vi "Calculate Average Center.vi"(11 "Gantry Fiducials":dbl[](array[numeric])) -> (1 "Sensor ID Location":dbl[](array[numeric]), 2 "CH1 Location":dbl[](array[numeric]), 3 "XYZTheta":dbl[](array[numeric]))   [LabVIEW 2018, in "Component Tray.lvclass"]
uses:
  Component Tray.lvclass
  <vilib>/Analysis/baseanly.llb/Mean (DBL).vi
  <vilib>/Analysis/NI_AALBase.lvlib
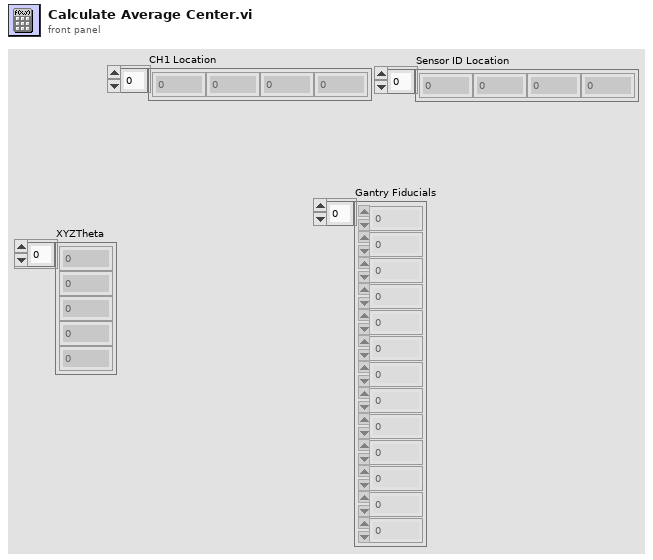
[diagram p1: front panel]
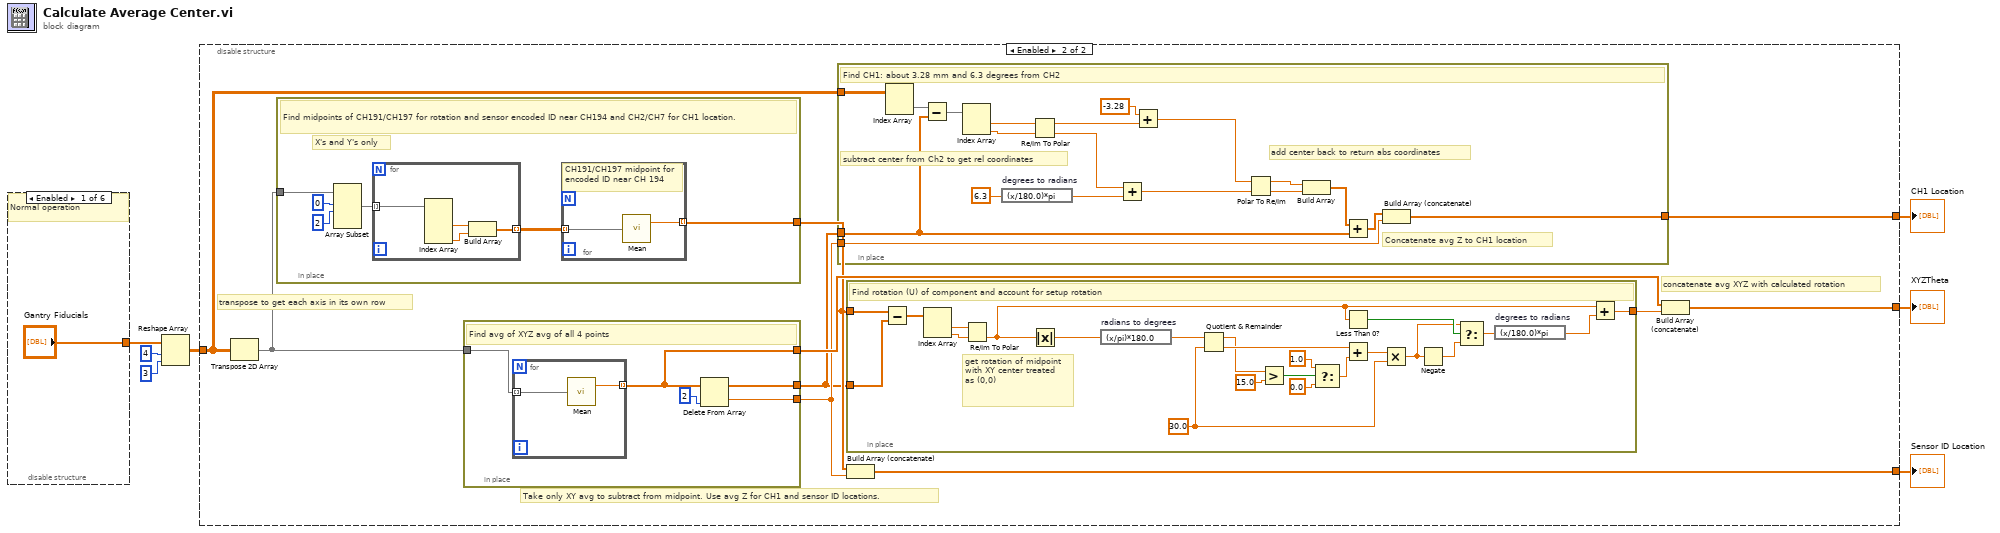
[diagram p0: block diagram]
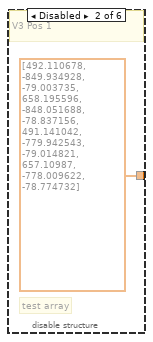
[diagram p2: hidden frame]
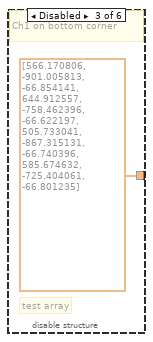
[diagram p3: hidden frame]
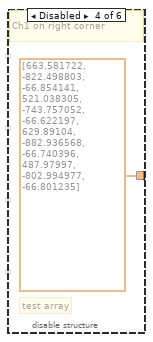
[diagram p4: hidden frame]
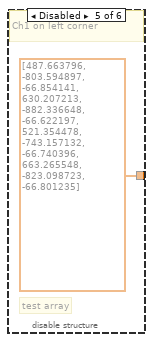
[diagram p5: hidden frame]
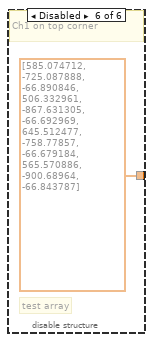
[diagram p6: hidden frame]
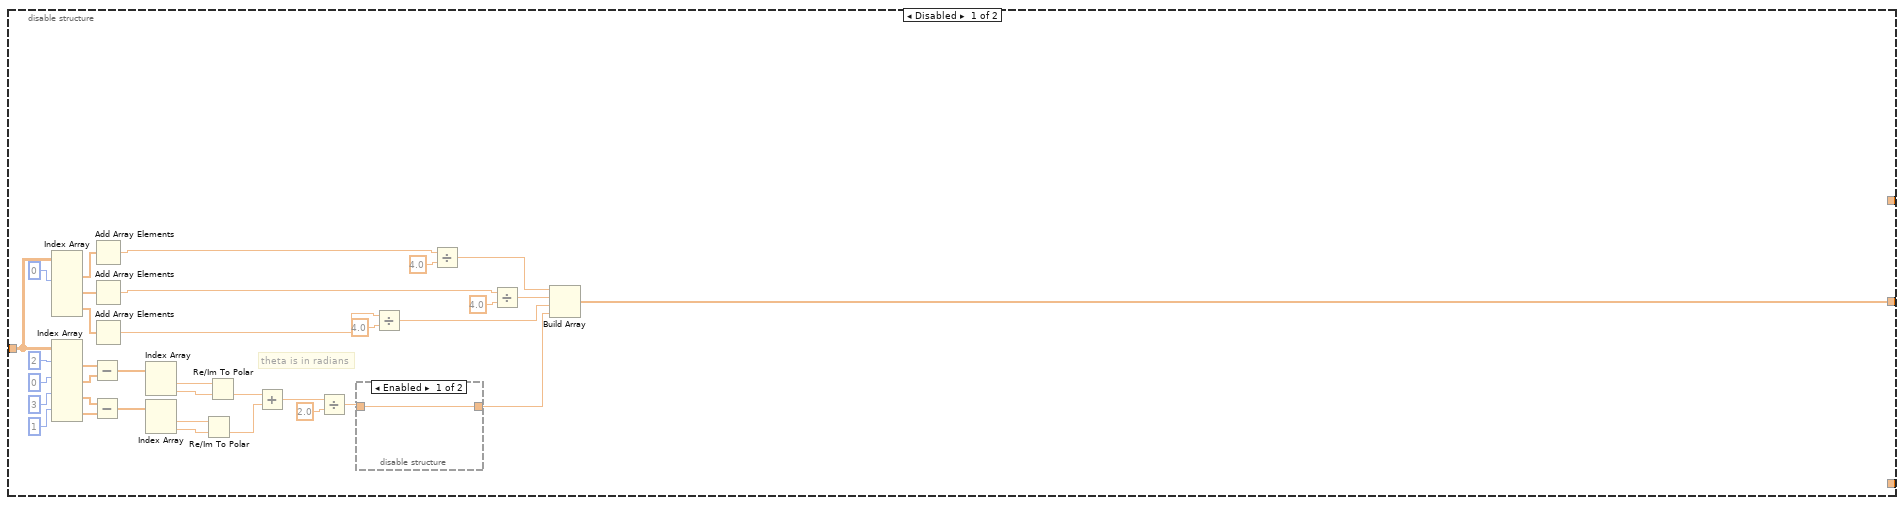
[diagram p7: hidden frame]
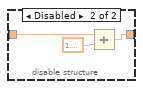
[diagram p8: hidden frame]
diagram:
  n1 = disable-structure shown="Enabled" {
    disable-tunnel: ["Gantry Fiducials" dbl[] [492.110678, -849.934928, -79.003735, 658.195596, -848.051688, -78.837156, 491.141042, -779.942543, -79.014821, 657.10987, -778.009622, -78.774732] dbl[] [566.170806, -901.005813, -66.854141, 644.912557, -758.462396, -66.622197, 505.733041, -867.315131, -66.740396, 585.674632, -725.404061, -66.801235] dbl[] [663.581722, -822.498803, -66.854141, 521.038305, -743.757052, -66.622197, 629.89104, -882.936568, -66.740396, 487.97997, -802.994977, -66.801235] dbl[] [487.663796, -803.594897, -66.854141, 630.207213, -882.336648, -66.622197, 521.354478, -743.157132, -66.740396, 663.265548, -823.098723, -66.801235] dbl[] [585.074712, -725.087888, -66.890846, 506.332961, -867.631305, -66.692969, 645.512477, -758.77857, -66.679184, 565.570886, -900.68964, -66.843787]] -> w6
    frame Enabled {
      # "Normal operation"
    }
    frame Disabled {
      # "test array"
      # "V3 Pos 1"
    }
    frame Disabled {
      # "test array"
      # "Ch1 on bottom corner"
    }
    frame Disabled {
      # "test array"
      # "Ch1 on right corner"
    }
    frame Disabled {
      # "test array"
      # "Ch1 on left corner"
    }
    frame Disabled {
      # "test array"
      # "Ch1 on top corner"
    }
  }
  n2 = Reshape Array(w6, 4 ("dimension size"), 3 ("dimension size")) -> (w3:dbl[][])
  n3 = disable-structure shown="Enabled" {
    disable-tunnel: [w18 w62] -> w7
    disable-tunnel: w3 -> [w17 w53]
    disable-tunnel: [_ w58] -> w5
    disable-tunnel: [_ w61] -> w4
    frame Disabled {
      # "theta is in radians"
      n4 = Index Array(array=w17, index (col) #1=0 ("disabled index (col)")) -> (element #1=w47:dbl[], element #2=w46:dbl[], element #3=w16:dbl[])  [unwired: 5 in]
      n5 = Index Array(array=w17, index (row) #1=2 ("index (row)"), index (row) #2=0 ("index (row)"), index (row) #3=3 ("index (row)"), index (row) #4=1 ("index (row)")) -> (element #1=w31:dbl[], element #2=w30:dbl[], element #3=w29:dbl[], element #4=w28:dbl[])  [unwired: 4 in]
      n6 = Subtract(x=w31, y=w30) -> (x-y=w41:dbl[])
      n7 = Subtract(x=w29, y=w28) -> (x-y=w40:dbl[])
      n8 = Add Array Elements(numeric array=w47) -> (sum=w45:dbl)
      n9 = Add Array Elements(numeric array=w46) -> (sum=w44:dbl)
      n10 = Add Array Elements(numeric array=w16) -> (sum=w22:dbl)
      n11 = Index Array(array=w41) -> (element #1=w39:dbl, element #2=w38:dbl)  [unwired: 2 in]
      n12 = Index Array(array=w40) -> (element #1=w37:dbl, element #2=w36:dbl)  [unwired: 2 in]
      n13 = Re/Im To Polar(2:w36, 3:w37) -> (0:w34:dbl)  [unwired: 1 out]
      n14 = Re/Im To Polar(2:w38, 3:w39) -> (0:w35:dbl)  [unwired: 1 out]
      n15 = Add(x=w35, y=w34) -> (x+y=w33:dbl)
      n16 = Divide(x=w33, y=2.0) -> (x/y=w15:dbl)
      n17 = disable-structure shown="Enabled" {
        disable-tunnel: w15 -> [w49 w51]
        disable-tunnel: [w49 w50] -> w14
        frame Enabled {
        }
        frame Disabled {
          n18 = Add(x=w51, y=1.5707963267948966) -> (x+y=w50:dbl)
        }
      }
      n19 = Divide(x=w22, y=4.0) -> (x/y=w19:dbl)
      n20 = Divide(x=w45, y=4.0) -> (x/y=w21:dbl)
      n21 = Divide(x=w44, y=4.0) -> (x/y=w20:dbl)
      n22 = Build Array(w21, w20, w19, w14) -> (w18:dbl[])
    }
    frame Enabled {
      # "concatenate avg XYZ with calculated rotation"
      # "Take only XY avg to subtract from midpoint. Use avg Z for CH1 and sensor ID locations."
      # "transpose to get each axis in its own row"
      n23 = Transpose 2D Array(2D array=w53) -> (transposed array=w59:dbl[][])
      n24 = in-place {
        in-place-border: w59 -> [w110]
        in-place-border: [w105] -> w56
        # "X's and Y's only"
        # "Find midpoints of CH191/CH197 for rotation and sensor encoded ID near CH194 and CH2/CH7 for CH1 location."
        n25 = Array Subset(array=w110, index (row)=0 ("index"), length (row)=2 ("length")) -> (w107:dbl[][])  [unwired: 2 in]
        n26 = for {
          tunnel: w107 -> [w116] mode=indexing
          tunnel: [w113] -> w106 mode=indexing
          n27 = Index Array(array=w116) -> (element #2=w115:dbl, element #4=w114:dbl)  [unwired: 4 in, 2 out]
          n28 = Build Array(w115, w114) -> (w113:dbl[])
        }
        n29 = for {
          tunnel: [w111] -> w105 mode=indexing
          tunnel: w106 -> [w112] mode=indexing
          # "CH191/CH197 midpoint for encoded ID near CH 194"
          n30 = call-poly <vilib>:"Mean.vi"("X"=w112) -> ("mean"=w111:dbl)  [unwired: 1 out]
        }
      }
      n31 = in-place {
        in-place-border: w59 -> [w121]
        in-place-border: [w120] -> w60
        in-place-border: [w118] -> w57
        in-place-border: [w117] -> w55
        # "Find avg of XYZ avg of all 4 points"
        n32 = for {
          tunnel: [w123] -> w120 mode=indexing
          tunnel: w121 -> [w122] mode=indexing
          n33 = call-poly <vilib>:"Mean.vi"("X"=w122) -> ("mean"=w123:dbl)  [unwired: 1 out]
        }
        n34 = Delete From Array(array=w120, index=2) -> (deleted portion=w118:dbl, array with subset deleted=w117:dbl[])  [unwired: 1 in]
      }
      n35 = in-place {
        in-place-border: w55 -> [w65]
        in-place-border: w57 -> [w64]
        in-place-border: [w81] -> w58
        in-place-border: w53 -> [w79]
        # "add center back to return abs coordinates"
        # "subtract center from Ch2 to get rel coordinates"
        # "Concatenate avg Z to CH1 location"
        # "Find CH1: about 3.28 mm and 6.3 degrees from CH2"
        n36 = Index Array(array=w79) -> (element=w80:dbl[])  [unwired: 2 in]
        n37 = Subtract(x=w80, y=w65) -> (x-y=w78:dbl[])
        n38 = Index Array(array=w78) -> (element #1=w77:dbl, element #2=w76:dbl)  [unwired: 2 in]
        n39 = expression code="(x/180.0)*pi" "degrees to radians"(6.3) -> (w70:dbl)
        n40 = Re/Im To Polar(2:w76, 3:w77) -> (0:w71:dbl, 1:w74:dbl)
        n41 = Add(x=w71, y=w70) -> (x+y=w69:dbl)
        n42 = Add(x=-3.28 ("r"), y=w74) -> (x+y=w72:dbl)
        n43 = Polar To Re/Im(2:w69, 3:w72) -> (0:w67:dbl, 1:w68:dbl)
        n44 = Build Array(w68, w67) -> (w66:dbl[])
        n45 = Add(x=w66, y=w65) -> (x+y=w63:dbl[])
        n46 = Build Array (concatenate)(w63, w64) -> (w81:dbl[])
      }
      n47 = in-place {
        in-place-border: w55 -> [w101]
        in-place-border: w56 -> [w100]
        in-place-border: [w99] -> w54
        w84 = 30.0 ("y")
        # "get rotation of midpoint with XY center treated as (0,0)"
        # "Find rotation (U) of component and account for setup rotation"
        n48 = Subtract(x=w100, y=w101) -> (x-y=w102:dbl[])
        n49 = Index Array(array=w102) -> (element #1=w103:dbl, element #2=w104:dbl)  [unwired: 2 in]
        n50 = Re/Im To Polar(2:w104, 3:w103) -> (0:w83:dbl)  [unwired: 1 out]
        n51 = Absolute Value(x=w83) -> (abs(x)=w82:dbl)
        n52 = expression code="(x/pi)*180.0" "radians to degrees"(w82) -> (w96:dbl)
        n53 = Quotient & Remainder(x=w96, y=w84) -> (x-y*floor(x/y)=w89:dbl, floor(x/y)=w92:dbl)
        n54 = Greater?(x=w89, y=15.0) -> (0:w90:bool)
        n55 = Select(t=1.0, s=w90, f=0.0) -> (s? t:f=w91:dbl)
        n56 = Less Than 0?(x=w83) -> (x < 0?=w97:bool)
        n57 = Add(x=w92, y=w91) -> (x+y=w85:dbl)
        n58 = Multiply(x=w85, y=w84) -> (x*y=w94:dbl)
        n59 = Negate(x=w94) -> (-x=w95:dbl)
        n60 = Select(t=w94, s=w97, f=w95) -> (s? t:f=w93:dbl)
        n61 = expression code="(x/180.0)*pi" "degrees to radians"(w93) -> (w98:dbl)
        n62 = Add(x=w83, y=w98) -> (x+y=w99:dbl)
      }
      n63 = Build Array (concatenate)(w56, w57) -> (w61:dbl[])
      n64 = Build Array (concatenate)(w60, w54) -> (w62:dbl[])
    }
  }
  "XYZTheta" <- w7
  "CH1 Location" <- w5
  "Sensor ID Location" <- w4
